vi "Write SA Pin.vi"(8 "error in (no error)":errorcluster, 10 "SA Pin":string, 11 "GSM_PVT in":refnum<class "GSM_PVT.lvclass">=refnum) -> (0 "error out":errorcluster, 3 "GSM_PVT out":refnum<class "GSM_PVT.lvclass">)   [LabVIEW 2016, in "SeqAuto Evaluations.lvlib" / "GSM_PVT.lvclass"]
uses:
  GSM_PVT.lvclass
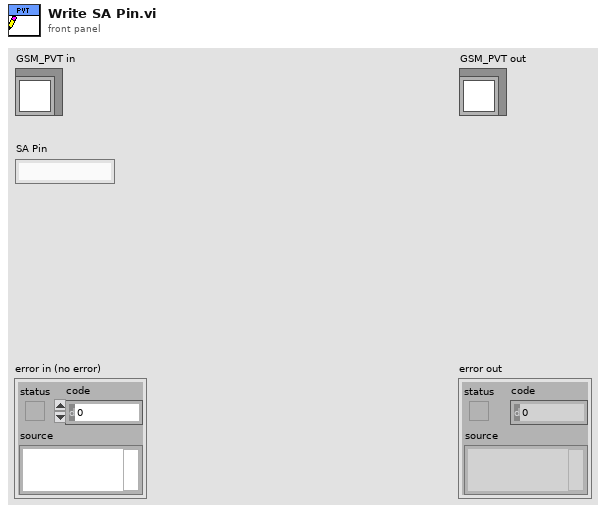
[diagram p1: front panel]
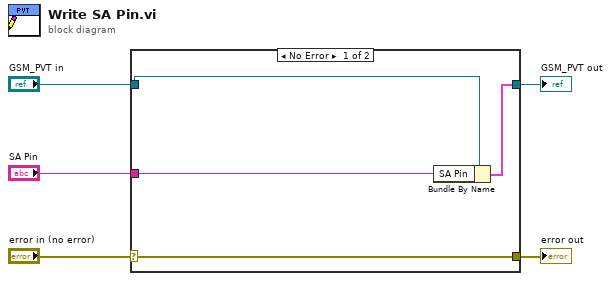
[diagram p0: block diagram]
diagram:
  n1 = case shown="No Error" "error in (no error)" {
    selector: "error in (no error)" -> [w9 w10]
    tunnel: [w9 w10] -> w4
    tunnel: [w7 w11] -> w2
    tunnel: "GSM_PVT in" -> [w8 w11]
    tunnel: "SA Pin" -> [w6 _]
    frame No Error {
      n2 = Bundle By Name(cluster=w8, "SA Pin"=w6) -> (w7:cluster{})
    }
    frame Error {
    }
  }
  "error out" <- w4
  "GSM_PVT out" <- w2
